vi "Send Command (non-enum).vi"(8 "error in (no error)":errorcluster, 10 "Commands":string[](array[string]), 11 "Gen 2 in":refnum<class "Gen 2.lvclass">) -> (0 "error out":errorcluster, 3 "Gen 2 out":refnum<class "Gen 2.lvclass">)   [LabVIEW 2018, in "Gen 2.lvlib" / "Gen 2.lvclass"]
doc: "This Override can send multiple commands that do not require a response from the targeted device."
uses:
  Gen 2.lvclass
  PPLs/Laser/Parent/Laser.lvlibp/Laser.lvclass
  C:/Projects/LabVIEW/PPLs/Laser/Parent/Laser.lvlibp/Laser.lvclass
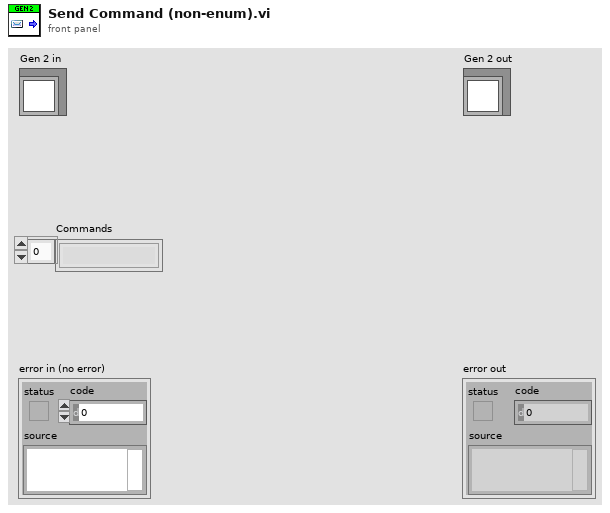
[diagram p1: front panel]
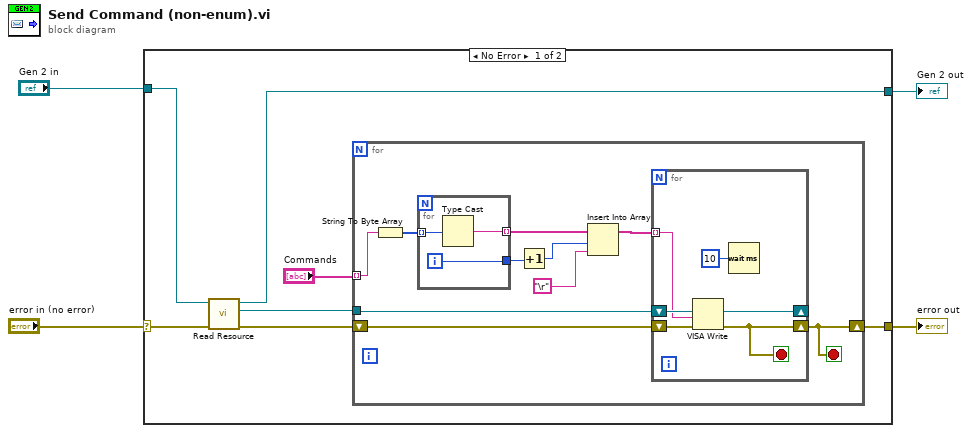
[diagram p0: block diagram]
diagram:
  n1 = case shown="No Error" "error in (no error)" {
    selector: "error in (no error)" -> [w11 w31]
    tunnel: "Gen 2 in" -> [w10 w32]
    tunnel: [w7 w32] -> w2
    tunnel: [w6 w31] -> w1
    frame No Error {
      n2 = call "Read Resource.vi"("error in (no error)"=w11, "Laser in"=w10) -> ("error out"=w9:errorcluster, "Resource"=w5:refnum<visa-resource-name>, "Laser out"=w7:refnum<class "Gen 2.lvclass">)  [unwired: 7 in]
      n3 = for {
        shift-right: [w19] -> w6
        shift-left: w9 -> [w20]
        tunnel: w5 -> [w21]
        tunnel: "Commands" -> [w18] mode=indexing
        stop <- w19 stop-if-true
        n4 = String To Byte Array(string=w18) -> (unsigned byte array=w17:u8[])
        n5 = for {
          tunnel: w17 -> [w30] mode=indexing
          tunnel: [w29] -> w15 mode=indexing
          tunnel: [w28] -> w16
          i -> [w28]
          n6 = Type Cast(x=w30) -> (*(type *) &x=w29:string)  [unwired: 1 in]
        }
        n7 = Increment(x=w16) -> (x+1=w14:i32)
        n8 = Insert Into Array(array=w15, index=w14, new element="\r") -> (w13:string[])
        n9 = for {
          shift-right: [w22] -> w19
          shift-left: w20 -> [w26]
          tunnel: w13 -> [w25] mode=indexing
          shift-right: [w24] -> _
          shift-left: w21 -> [w27]
          stop <- w22 stop-if-true
          n10 = VISA Write(VISA resource name=w27, write buffer=w25, error in (no error)=w26) -> (VISA resource name out=w24:refnum<visa-resource-name>, error out=w22:errorcluster)  [unwired: 1 out]
          n11 = Wait (ms)(milliseconds to wait=u32 10) -> ()  [unwired: 1 out]
        }
      }
    }
    frame Error {
    }
  }
  "error out" <- w1
  "Gen 2 out" <- w2
